vi "CSUMetClient.vi"() -> (0 "Time Of Value (s)":dbl format="%#.1f", 1 "Error":bool, 2 "RawPressure/mBar":dbl)   [LabVIEW 2018]
uses:
  <vilib>/httpClient/LabVIEWHTTPClient.lvlib
panel:
  out "ComputerTime":timestamp
  out "MetTimeStamp":timestamp
  out "data out":string
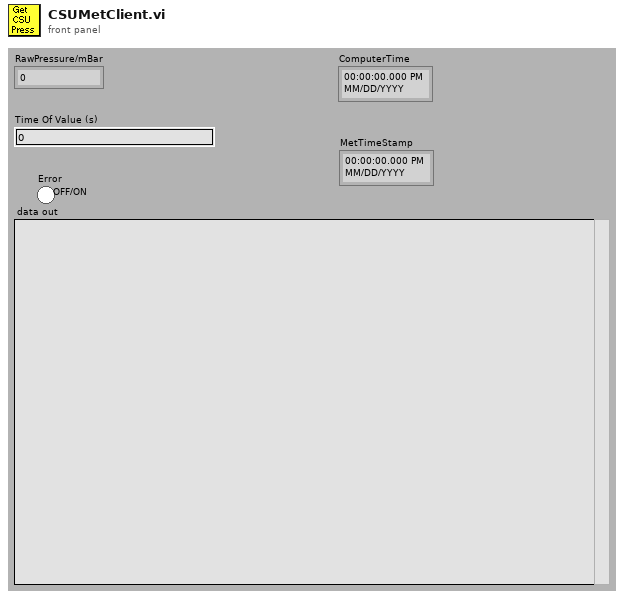
[diagram p1: front panel]
types:
  T1 = typedef "LabVIEWHTTPClient.lvlib/ClientHandle.ctl" = refnum<k1>
  T2 = cluster{"second":i32, "minute":i32, "hour":i32, "day of month":i32, "month":i32, "year":i32, "day of week":i32, "day of year":i32, "is DST":i32}
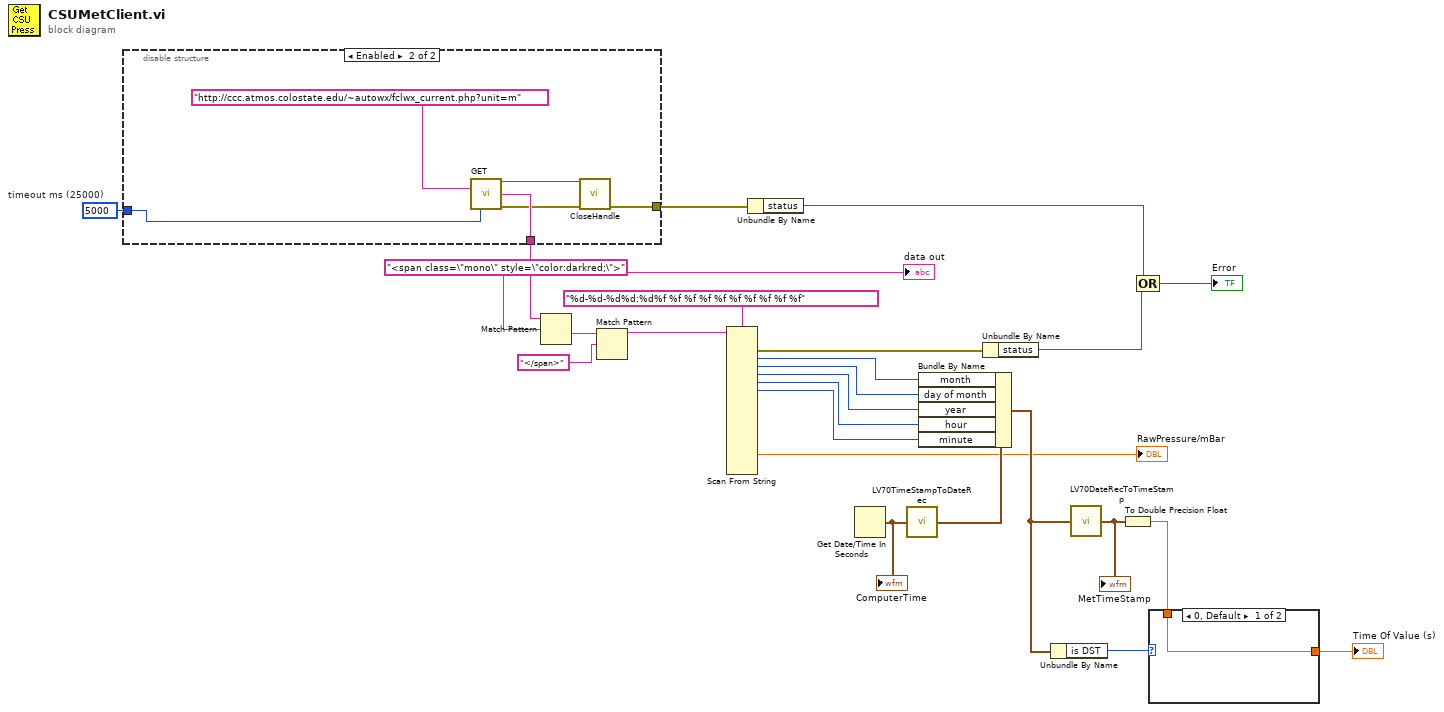
[diagram p0: block diagram]
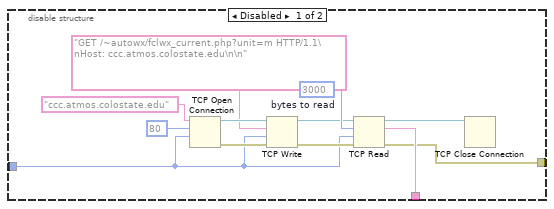
[diagram p2: hidden frame]
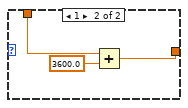
[diagram p3: hidden frame]
diagram:
  w2 = 5000  # timeout ms (25000)
  n1 = disable-structure shown="Enabled" {
    disable-tunnel: [w28 w43] -> w13
    disable-tunnel: w2 -> [w27 w42]
    disable-tunnel: [w26 w38] -> w1
    frame Disabled {
      w30 = 3000  # bytes to read
      n2 = TCP Open Connection(address="ccc.atmos.colostate.edu", remote port or service name=u16 80 ("remote port"), timeout ms (60000)=w27) -> (connection ID=w35:refnum<k5>, error out=w33:errorcluster)  [unwired: 1 in, 1 out]
      n3 = TCP Write(connection ID=w35, data in="GET /~autowx/fclwx_current.php?unit=m HTTP/1.1\nHost: ccc.atmos.colostate.edu\n\n", error in (no error)=w33, 9:w27) -> (connection ID out=w29:refnum<k5>, error out=w32:errorcluster)  [unwired: 1 out]
      n4 = TCP Read(connection ID=w29, bytes to read=w30, error in (no error)=w32, 9:w27) -> (connection ID out=w31:refnum<k5>, data out=w28:string, error out=w26:errorcluster)  [unwired: 1 out]
      n5 = TCP Close Connection(connection ID=w31) -> ()  [unwired: 1 in, 3 out]
    }
    frame Enabled {
      n6 = call <vilib>:"GET.vi"("url"="http://ccc.atmos.colostate.edu/~autowx/fclwx_current.php?unit=m", "timeout (10000)"=w42) -> ("client handle out"=w40:T1, "body"=w43:string, "error out"=w39:errorcluster)  [unwired: 10 in, 1 out]
      n7 = call <vilib>:"CloseHandle.vi"("client handle"=w40, "error in (no error)"=w39) -> ("error out"=w38:errorcluster)  [unwired: 13 in]
    }
  }
  "data out" <- w13
  n8 = Match Pattern(string=w13, regular expression="<span class=\"mono\" style=\"color:darkred;\">") -> (after substring=w15:string)  [unwired: 4 out]
  n9 = Match Pattern(string=w15, regular expression="</span>") -> (before substring=w12:string)  [unwired: 4 out]
  n10 = Scan From String(format string="%d-%d-%d%d:%d%f %f %f %f %f %f %f %f %f %f", input string=w12) -> (error out=w9:errorcluster, output 1=w4:i32, output 2=w5:i32, output 3=w6:i32, output 4=w7:i32, output 5=w8:i32, output 13=→"RawPressure/mBar":dbl)  [unwired: 2 in, 26 out]
  n11 = Unbundle By Name(w1) -> ("status"=w20:bool)
  n12 = Get Date/Time In Seconds() -> (seconds since 1Jan1904=w17:timestamp)
  "ComputerTime" <- w17
  n13 = call <vilib>:"LV70TimeStampToDateRec.vi"("time stamp"=w17) -> ("date time rec"=w25:T2)
  n14 = Bundle By Name(cluster=w25, "month"=w4, "day of month"=w5, "year"=w6, "hour"=w7, "minute"=w8) -> (w23:T2)
  n15 = Unbundle By Name(w9) -> ("status"=w10:bool)
  n16 = Unbundle By Name(w23) -> ("is DST"=w22:i32)
  n17 = call <vilib>:"LV70DateRecToTimeStamp.vi"("date time rec"=w23) -> ("Time Stamp"=w24:timestamp)
  "MetTimeStamp" <- w24
  n18 = To Double Precision Float(number=w24) -> (double precision float=w21:dbl)
  n19 = Compound Arithmetic op=OR(w20, w10) -> (→"Error":bool)
  n20 = case shown="0, Default" w22 {
    tunnel: w21 -> [w44 w47]
    tunnel: [w44 w45] -> w18
    frame 0, Default {
    }
    frame 1 {
      n21 = Add(x=w47, y=3600.0) -> (x+y=w45:dbl)
    }
  }
  "Time Of Value (s)" <- w18
